vi "Servo3.vi"() -> ()   [LabVIEW 2013]
uses:
  <vilib>/LabVIEW Interface for Arduino/LabVIEW Interface for Arduino.lvlib
panel:
  in  "Pin Servo":u8=2
  out "Valor PWM":u8(knob) scale=0.0..180.0
  in  "Consigna":dbl(knob) scale=0.0..180.0
  in  "stop":bool
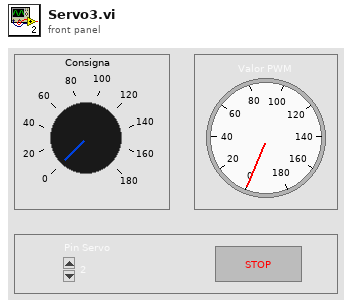
[diagram p1: front panel]
types:
  T1 = typedef "LabVIEW Interface for Arduino.lvlib/Arduino Resource.ctl" = cluster{"VISA resource":refnum<visa-resource-name>, "Board Type":T2, "Connection Type":enum8{"USB / Serial"}, "Bytes Per Packet (15)":u8}
  T2 = typedef "LabVIEW Interface for Arduino.lvlib/Board Type.ctl" = enum16{"Uno", "Dimuelanove w/Atmega 328", "Mega 2560"}
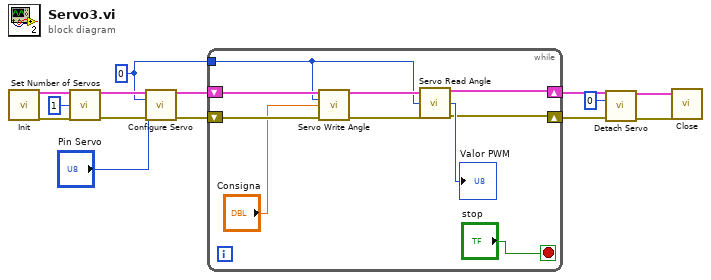
[diagram p0: block diagram]
diagram:
  w7 = u8 0 ("Servo Number (0)")
  n1 = call <vilib>:"Init.vi"() -> ("Arduino Resource"=w14:T1, "error out"=w13:errorcluster)  [unwired: 18 in]
  n2 = call <vilib>:"Set Number of Servos.vi"("Arduino Resource"=w14, "Number Of Servos (1)"=u8 1, "error in"=w13) -> ("Arduino Resource"=w10:T1, "error out"=w11:errorcluster)  [unwired: 11 in]
  n3 = call <vilib>:"Configure Servo.vi"("Arduino Resource"=w10, "Servo Number (0)"=w7, "DIO Pin (2)"="Pin Servo", "error in"=w11) -> ("Arduino Resource"=w9:T1, "error out"=w8:errorcluster)  [unwired: 10 in]
  n4 = while {
    tunnel: w7 -> [w15]
    shift-right: [w18] -> w6
    shift-left: w9 -> [w22]
    shift-right: [w17] -> w5
    shift-left: w8 -> [w23]
    stop <- "stop" stop-if-true
    n5 = call <vilib>:"Servo Write Angle.vi"("Arduino Resource"=w22, "Servo Number"=w15, "Angle (Degrees)"="Consigna", "error in"=w23) -> ("Arduino Resource"=w21:T1, "error out"=w20:errorcluster)  [unwired: 10 in]
    n6 = call <vilib>:"Servo Read Angle.vi"("Arduino Resource"=w21, "Servo Number"=w15, "error in"=w20) -> ("Arduino Resource"=w18:T1, "Angle (Degrees)"=→"Valor PWM":u8, "error out"=w17:errorcluster)  [unwired: 10 in]
  }
  n7 = call <vilib>:"Detach Servo.vi"("Arduino Resource"=w6, "Servo Number"=u8 0, "error in"=w5) -> ("Arduino Resource"=w3:T1, "error out"=w4:errorcluster)  [unwired: 11 in]
  n8 = call <vilib>:"Close.vi"("Arduino Resource"=w3, "error in"=w4) -> ()  [unwired: 13 in, 1 out]
